vi "Sets the test name for AUTO.vi"(5 "Enable to Query":bool, 7 "Enable to Setup":bool, 8 "error in":errorcluster, 10 "Test name":string, 11 "VISA resource name":refnum<visa-resource-name>) -> (0 "error out":errorcluster, 2 "Return the test name":string, 3 "VISA resource name out":refnum<visa-resource-name>)   [LabVIEW 2011, in "GPT-9000.lvlib"]
uses:
  <instrlib>/GPT-9000/GPT-9000.lvlib
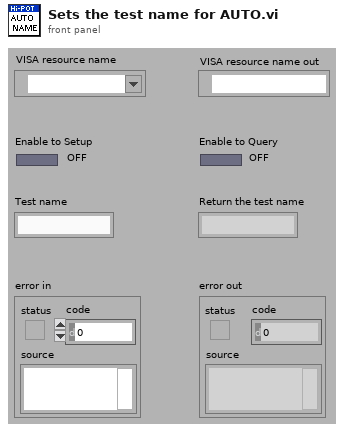
[diagram p1: front panel]
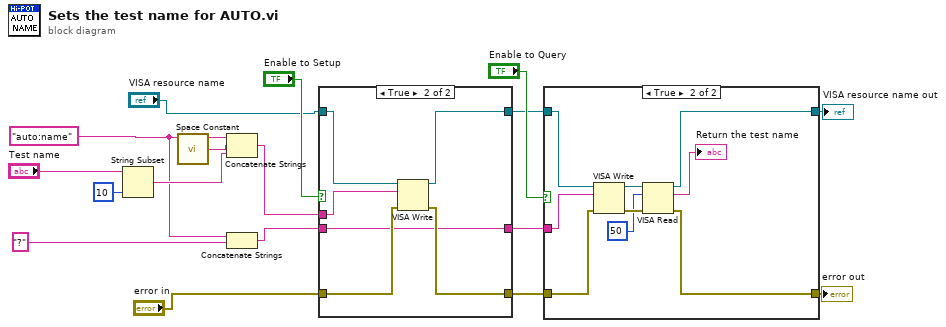
[diagram p0: block diagram]
diagram:
  w12 = "auto:name"
  n1 = String Subset(string="Test name", length (rest)=10 ("length (rest)")) -> (substring=w14:string)  [unwired: 1 in]
  n2 = call <vilib>:"Space Constant.vi"() -> ("String"=w15:string)
  n3 = Concatenate Strings(w12, w15, w14) -> (w10:string)
  n4 = Concatenate Strings(w12, "?") -> (w9:string)
  n5 = case shown="True" "Enable to Setup" {
    tunnel: w10 -> [_ w22]
    tunnel: w9 -> [w18 w21]
    tunnel: "VISA resource name" -> [w20 w26]
    tunnel: "error in" -> [w19 w25]
    tunnel: [w20 w24] -> w5
    tunnel: [w19 w23] -> w4
    tunnel: [w18 w21] -> w3
    frame False {
    }
    frame True {
      n6 = VISA Write(VISA resource name=w26, write buffer=w22, error in (no error)=w25) -> (VISA resource name out=w24:refnum<visa-resource-name>, error out=w23:errorcluster)  [unwired: 1 out]
    }
  }
  n7 = case shown="True" "Enable to Query" {
    tunnel: w5 -> [w28 w33]
    tunnel: w4 -> [w27 w32]
    tunnel: w3 -> [_ w34]
    tunnel: [w28 w31] -> w2
    tunnel: [w27 w30] -> w1
    frame False {
    }
    frame True {
      n8 = VISA Write(VISA resource name=w33, write buffer=w34, error in (no error)=w32) -> (VISA resource name out=w36:refnum<visa-resource-name>, error out=w37:errorcluster)  [unwired: 1 out]
      n9 = VISA Read(VISA resource name=w36, byte count=u32 50, error in (no error)=w37) -> (VISA resource name out=w31:refnum<visa-resource-name>, read buffer=→"Return the test name":string, error out=w30:errorcluster)  [unwired: 1 out]
    }
  }
  "VISA resource name out" <- w2
  "error out" <- w1
